vi "Stop Record.vi"(8 "error in (no error)":errorcluster, 11 "Spectrum Recorder in":refnum<class "Spectrum Recorder.lvclass">) -> (0 "error out":errorcluster, 3 "Spectrum Recorder out":refnum<class "Spectrum Recorder.lvclass">)   [LabVIEW 2016, in "Spectrum Recorder.lvclass"]
uses:
  Spectrum Recorder.lvclass
  Spectrum Recorder.lvclass/Spectrum Recorder.ctl
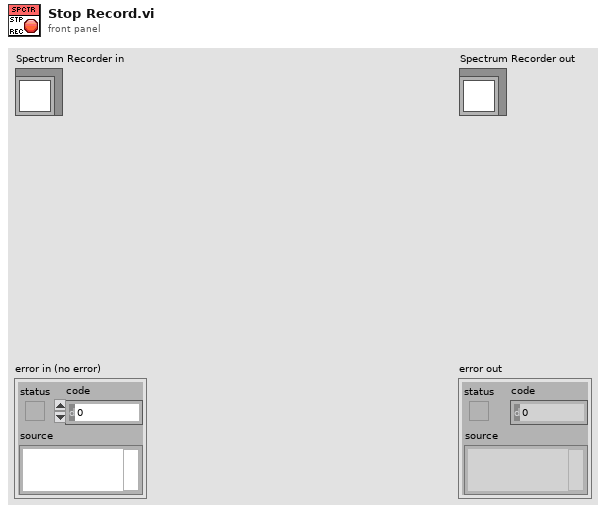
[diagram p1: front panel]
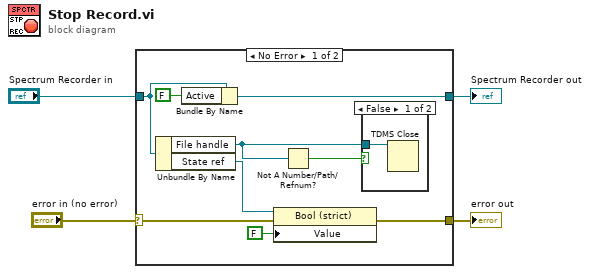
[diagram p0: block diagram]
diagram:
  n1 = case shown="No Error" "error in (no error)" {
    selector: "error in (no error)" -> [w13 w16]
    tunnel: [w7 w16] -> w3
    tunnel: [w12 w15] -> w1
    tunnel: "Spectrum Recorder in" -> [w11 w15]
    frame No Error {
      n2 = Unbundle By Name(w11) -> ("File handle"=w9:refnum<k34>, "State ref"=w5:refnum<vi>)
      n3 = Bundle By Name(cluster=w11, "Active"=FALSE) -> (w12:refnum<class "Spectrum Recorder.lvclass">)
      n4 = property class="Bool (strict)"(reference=w5, error in=w13, "Value"=FALSE) -> (error out=w7:errorcluster)  [unwired: 1 out]
      n5 = Not A Number/Path/Refnum?(number/path/refnum=w9) -> (NaN/Path/Refnum?=w10:bool)
      n6 = case shown="False" w10 {
        tunnel: w9 -> [w14 _]
        frame False {
          n7 = TDMS Close(11:w14) -> ()  [unwired: 1 in, 2 out]
        }
        frame True {
        }
      }
    }
    frame Error {
    }
  }
  "error out" <- w3
  "Spectrum Recorder out" <- w1
